vi "Set SMO.vi"(8 "error in (no error)":errorcluster, 10 "SMO.Template":refnum<class "SMO.Template.lvclass">, 11 "SMO.UI":refnum<class "SMO.UI.Template.lvclass">) -> (0 "error out":errorcluster, 3 "SMO.UI out":refnum<class "SMO.UI.Template.lvclass">)   [LabVIEW 2013, in "SMO.UI.Template.lvclass"]
doc: "Sets the SMO dependency."
uses:
  SMO.UI.Template.lvclass
  SMO.Template/SMO.Template.lvclass
  SMO.UI.Template.lvclass/SMO.UI.Template.ctl
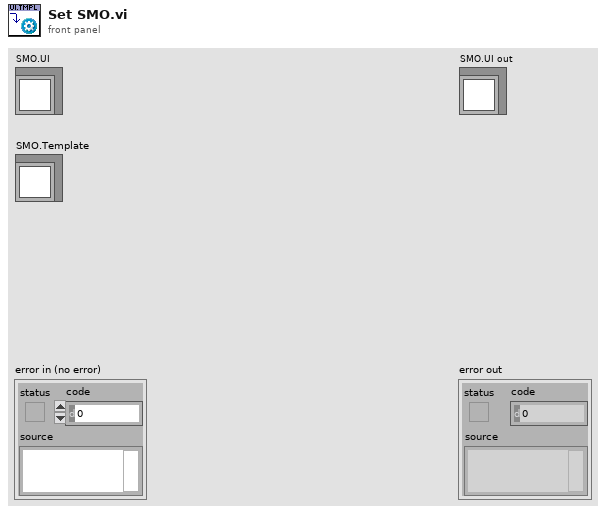
[diagram p1: front panel]
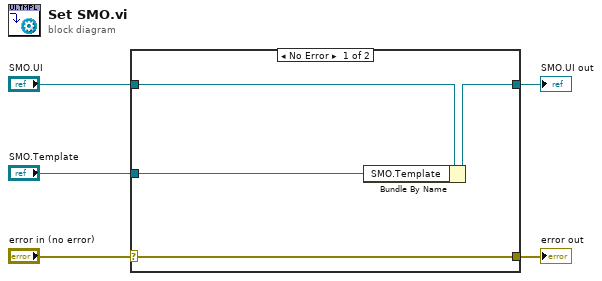
[diagram p0: block diagram]
diagram:
  n1 = case shown="No Error" "error in (no error)" {
    selector: "error in (no error)" -> [w9 w10]
    tunnel: [w9 w10] -> w4
    tunnel: [w6 w11] -> w2
    tunnel: "SMO.UI" -> [w8 w11]
    tunnel: "SMO.Template" -> [w7 _]
    frame No Error {
      n2 = Bundle By Name(cluster=w8, "SMO.Template"=w7) -> (w6:refnum<class "SMO.UI.Template.lvclass">)
    }
    frame Error {
    }
  }
  "error out" <- w4
  "SMO.UI out" <- w2
